vi "VHM-sendConnectionSettings.vi"(8 "error in (no error)":errorcluster, 11 "VHM-VNA_Hardware_Manager in":refnum<class "VHM-VNA_Hardware_Manager.lvclass">) -> (0 "error out":errorcluster, 3 "VHM-VNA_Hardware_Manager out":refnum<class "VHM-VNA_Hardware_Manager.lvclass">)   [LabVIEW 2020, in "VHM-VNA_Hardware_Manager.lvlib" / "VHM-VNA_Hardware_Manager.lvclass"]
uses:
  VHM-VNA_Hardware_Manager.lvclass
  VHM-connection_status.ctl
  VHM-VNA_Hardware_Manager.lvclass/VHM-VNA_Hardware_Manager.ctl
  VHMI-VNA_Hardware_manager_Interface Messages/VHMI-recieveConnectionInfo Msg/VHMI-recieveConnectionInfo Msg.lvclass/VHMI-recieveConnectionInfo Msg.ctl
  <vilib>/ActorFramework/Message Enqueuer/Message Enqueuer.lvclass/Message Enqueuer.ctl
  <vilib>/ActorFramework/Message Enqueuer/Enqueue.vi
  VHMI-VNA_Hardware_manager_Interface Messages/VHMI-recieveConnectionInfo Msg/VHMI-recieveConnectionInfo Msg.lvclass
  C:/Program Files (x86)/National Instruments/LabVIEW 2020/vi.lib/ActorFramework/Message/Message.lvclass
  <vilib>/ActorFramework/Message Priority Queue/Priority Enqueue.vi
  classes/vna-drivers/liteVNA/VD-LV-LiteVNA.lvclass
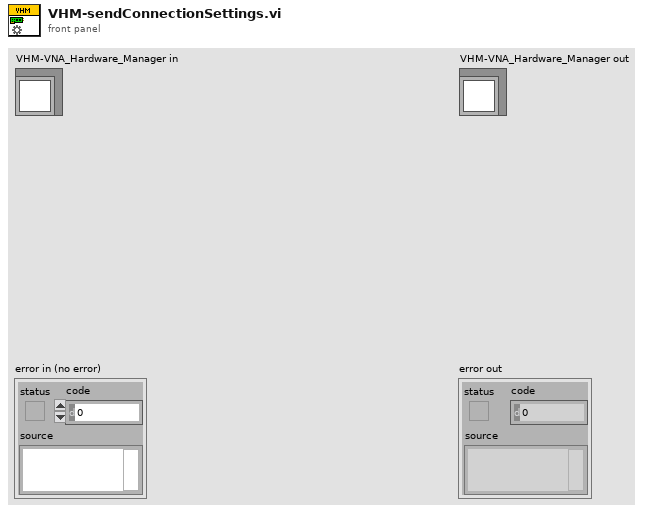
[diagram p1: front panel]
types:
  T1 = typedef "VHM-VNA_Hardware_Manager.lvlib/VHM-VNA_Hardware_Manager.lvclass/VHM-connection_status.ctl" = cluster{"Connected?":bool, "Status":string}
  T2 = typedef "VD-LV-LiteVNA.lvclass/VD-session_info.ctl" = cluster{"last set TS":timestamp, "last get TS":timestamp, "last set":T3, "last get":T3, "Connected?":bool}
  T3 = typedef "HP-S-Serial.lvclass/HP-S-data.ctl" = u8[]
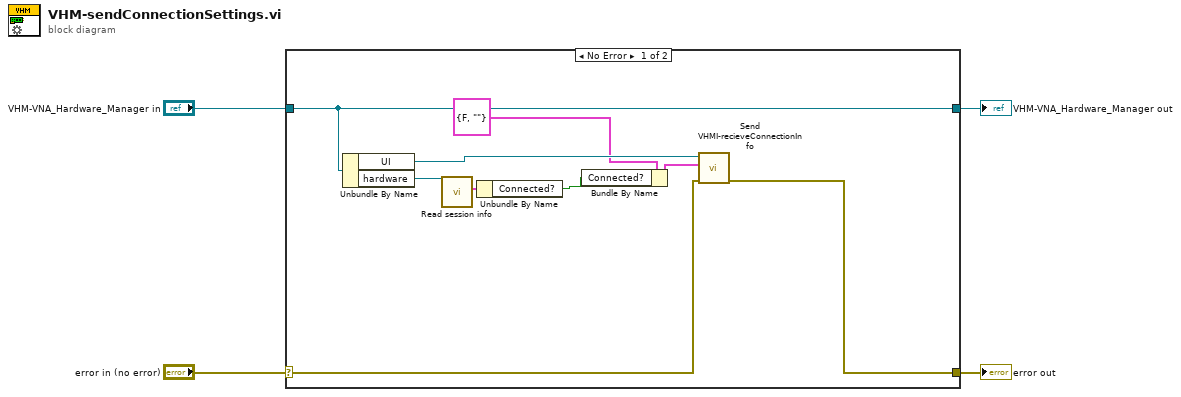
[diagram p0: block diagram]
diagram:
  n1 = case shown="No Error" "error in (no error)" {
    selector: "error in (no error)" -> [w5 w15]
    tunnel: [w6 w15] -> w3
    tunnel: [w13 w14] -> w1
    tunnel: "VHM-VNA_Hardware_Manager in" -> [w13 w14]
    frame No Error {
      n2 = Unbundle By Name(w13) -> ("UI"=w12:refnum<class "Message Enqueuer.lvclass">, "hardware"=w11:refnum<class "VD-LV-LiteVNA.lvclass">)
      n3 = call-dynamic "Read session info.vi"("VD-LV-LiteVNA in"=w11) -> ("session info"=w8:T2)  [unwired: 8 in, 2 out]
      n4 = Unbundle By Name(w8) -> ("Connected?"=w7:bool)
      n5 = Bundle By Name(cluster=T1 {"Connected?"=FALSE, "Status"=""} ("connection status"), "Connected?"=w7) -> (w9:T1)
      n6 = call "Send VHMI-recieveConnectionInfo.vi"("error in (no error)"=w5, "connection status"=w9, "Message Enqueuer"=w12) -> ("error out"=w6:errorcluster)  [unwired: 7 in, 1 out]
    }
    frame Error {
    }
  }
  "error out" <- w3
  "VHM-VNA_Hardware_Manager out" <- w1
